vi "Write InstrumentCommunication.vi"(8 "error in (no error)":errorcluster, 10 "InstrumentCommunication":string[][](array[string]), 11 "TestBench in":refnum<class "TestBench.lvclass">) -> (0 "error out":errorcluster, 3 "TestBench out":refnum<class "TestBench.lvclass">)   [LabVIEW 2019, in "TestBench.lvlib" / "TestBench.lvclass"]
uses:
  TestBench.lvclass
  TestBench.lvclass/TestBench.ctl
  TestEngine/TestEngine Messages/Write InstrumentCommunication Msg/Write InstrumentCommunication Msg.lvclass/Write InstrumentCommunication Msg.ctl
  <vilib>/ActorFramework/Message Enqueuer/Message Enqueuer.lvclass/Message Enqueuer.ctl
  <vilib>/ActorFramework/Message Enqueuer/Enqueue.vi
  TestEngine/TestEngine Messages/Write InstrumentCommunication Msg/Write InstrumentCommunication Msg.lvclass
  C:/Program Files (x86)/National Instruments/LabVIEW 2019/vi.lib/ActorFramework/Message/Message.lvclass
  <vilib>/ActorFramework/Message Priority Queue/Priority Enqueue.vi
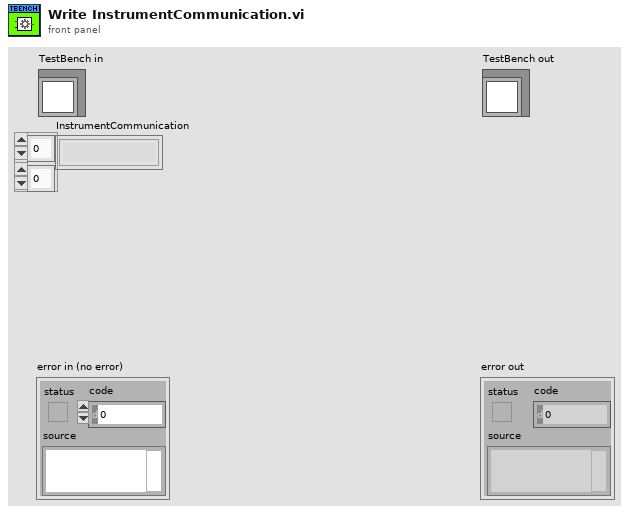
[diagram p1: front panel]
types:
  T1 = map{string, refnum<class "Message Enqueuer.lvclass">}
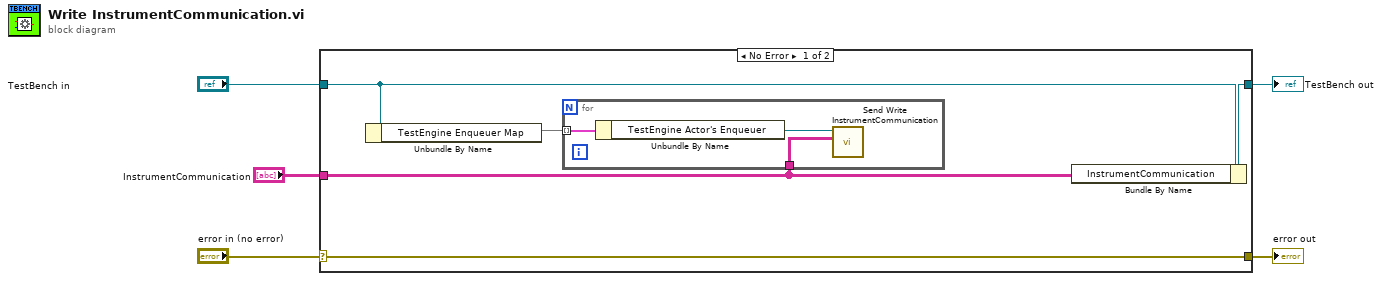
[diagram p0: block diagram]
diagram:
  n1 = case shown="No Error" "error in (no error)" {
    selector: "error in (no error)" -> [w10 w14]
    tunnel: [w10 w14] -> w4
    tunnel: [w9 w15] -> w2
    tunnel: "TestBench in" -> [w8 w15]
    tunnel: "InstrumentCommunication" -> [w6 _]
    frame No Error {
      n2 = Unbundle By Name(w8) -> ("TestEngine Enqueuer Map"=w7:T1)
      n3 = for {
        tunnel: w7 -> [w13] mode=indexing
        tunnel: w6 -> [w12]
        n4 = Unbundle By Name(w13) -> ("TestEngine Actor's Enqueuer"=w11:refnum<class "Message Enqueuer.lvclass">)
        n5 = call "Send Write InstrumentCommunication.vi"("InstrumentCommunication"=w12, "Message Enqueuer"=w11) -> ()  [unwired: 8 in, 2 out]
      }
      n6 = Bundle By Name(cluster=w8, "InstrumentCommunication"=w6) -> (w9:refnum<class "TestBench.lvclass">)
    }
    frame Error {
    }
  }
  "error out" <- w4
  "TestBench out" <- w2
